vi "TAT_Com_PLC.vi"() -> ()   [LabVIEW 2017]
uses:
  Controls/PLC_Comm_State.ctl
  <vilib>/NI/Modbus Library/API/Master/Modbus Master.lvclass
  C:/Program Files (x86)/National Instruments/LabVIEW 2017/vi.lib/NI/Modbus Library/API/Modbus API.lvclass
  <vilib>/NI/Modbus Library/API/Wrapper/Create TCP Master.vi
  Global/PLC_to_Auto.vi
  <vilib>/NI/Modbus Library/API/Modbus API.lvclass
  <vilib>/NI/Modbus Library/API/Wrapper/API Main.lvlib
panel:
  out "register values":u16[](array[numeric])
  out "Array 2":u16[](array[numeric])
  out "PREVIOUS STATE":T1
  out "PLC IP Address":string
  out "error out 2":errorcluster
  out "error IO":errorcluster
  in  "stop 2":bool
  out "PLC STATUS station 2":bool
  out "LIVE":errorcluster
  out "Latch Error Case":errorcluster
  in  "error in":errorcluster
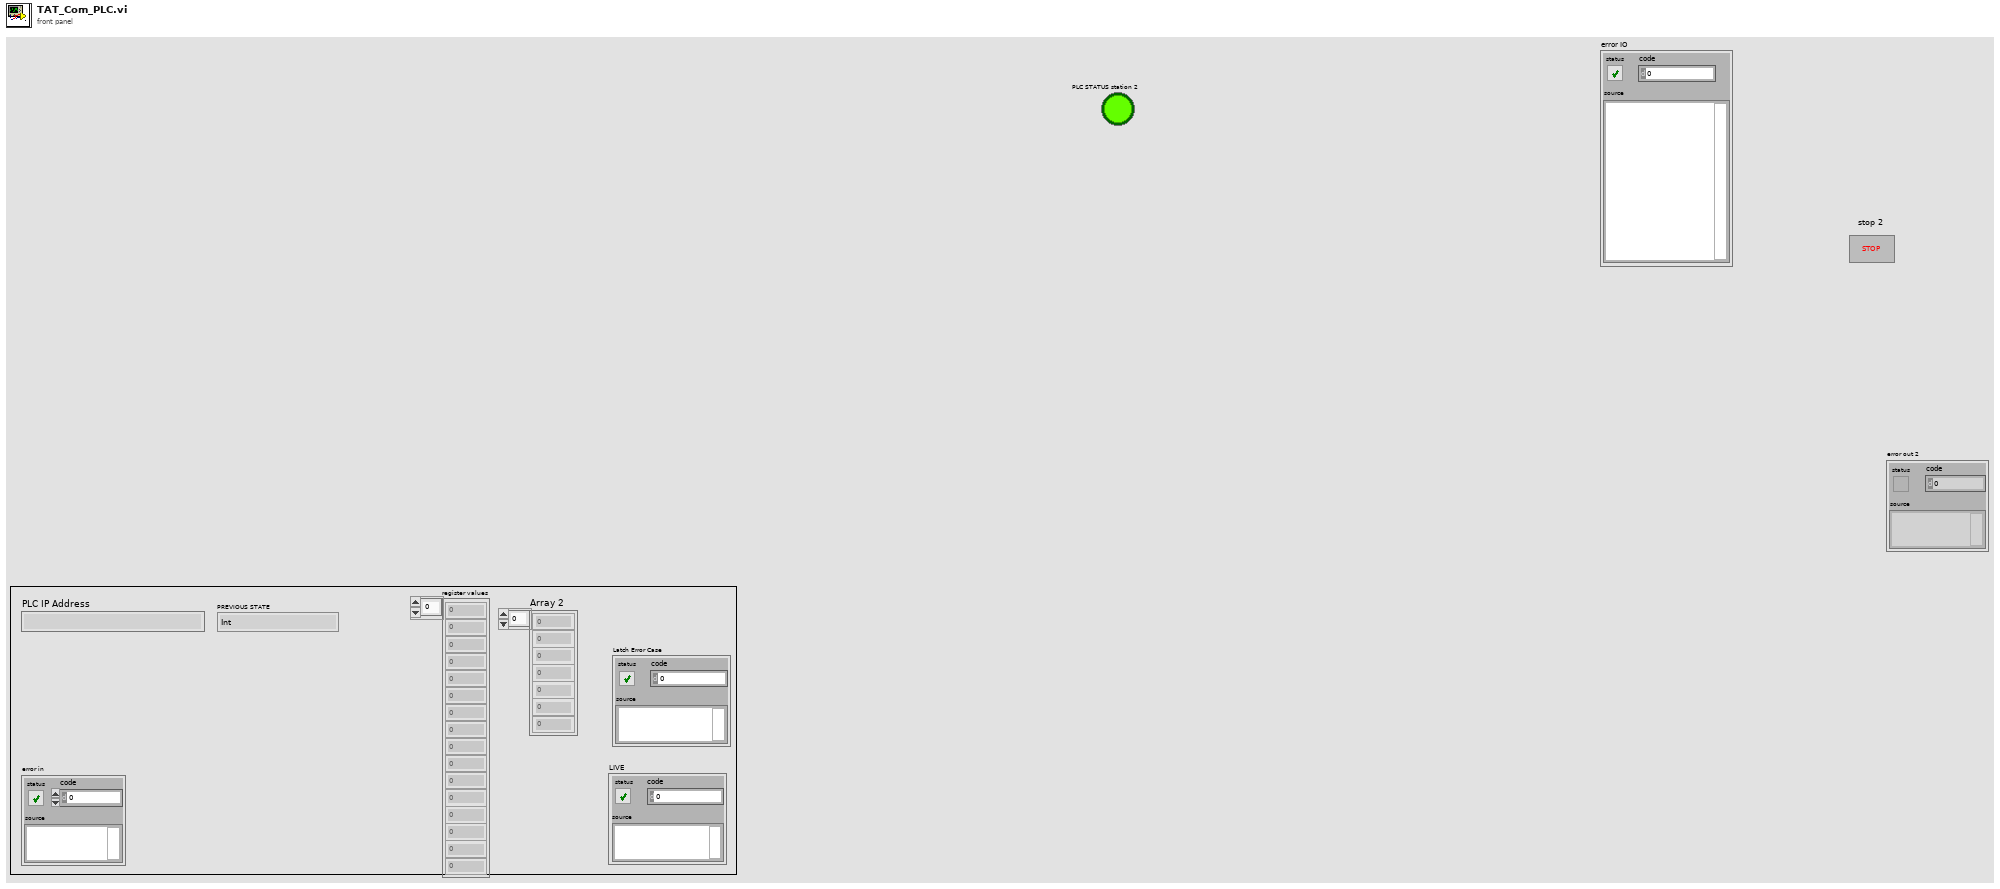
[diagram p1: front panel]
types:
  T1 = typedef "PLC_Comm_State.ctl" = enum16{"Int", "Connect", "Write", "Write2", "Write3", "Read", "Read2", "Read3", "Error", "Disconnect"}
  T2 = cluster{"PLC IP ADDRESS":string, "SCAN 1 COM":refnum<visa-resource-name>, "SCAN 2 COM":refnum<visa-resource-name>, "LOAD CELL COM":refnum<visa-resource-name>, "PRINTER IP ADDRESS":string}
  T3 = enum32{"invalid app kind", "Development System", "Run Time System", "Student Edition", "Embedded LabVIEW", "Evaluation", "Custom"}
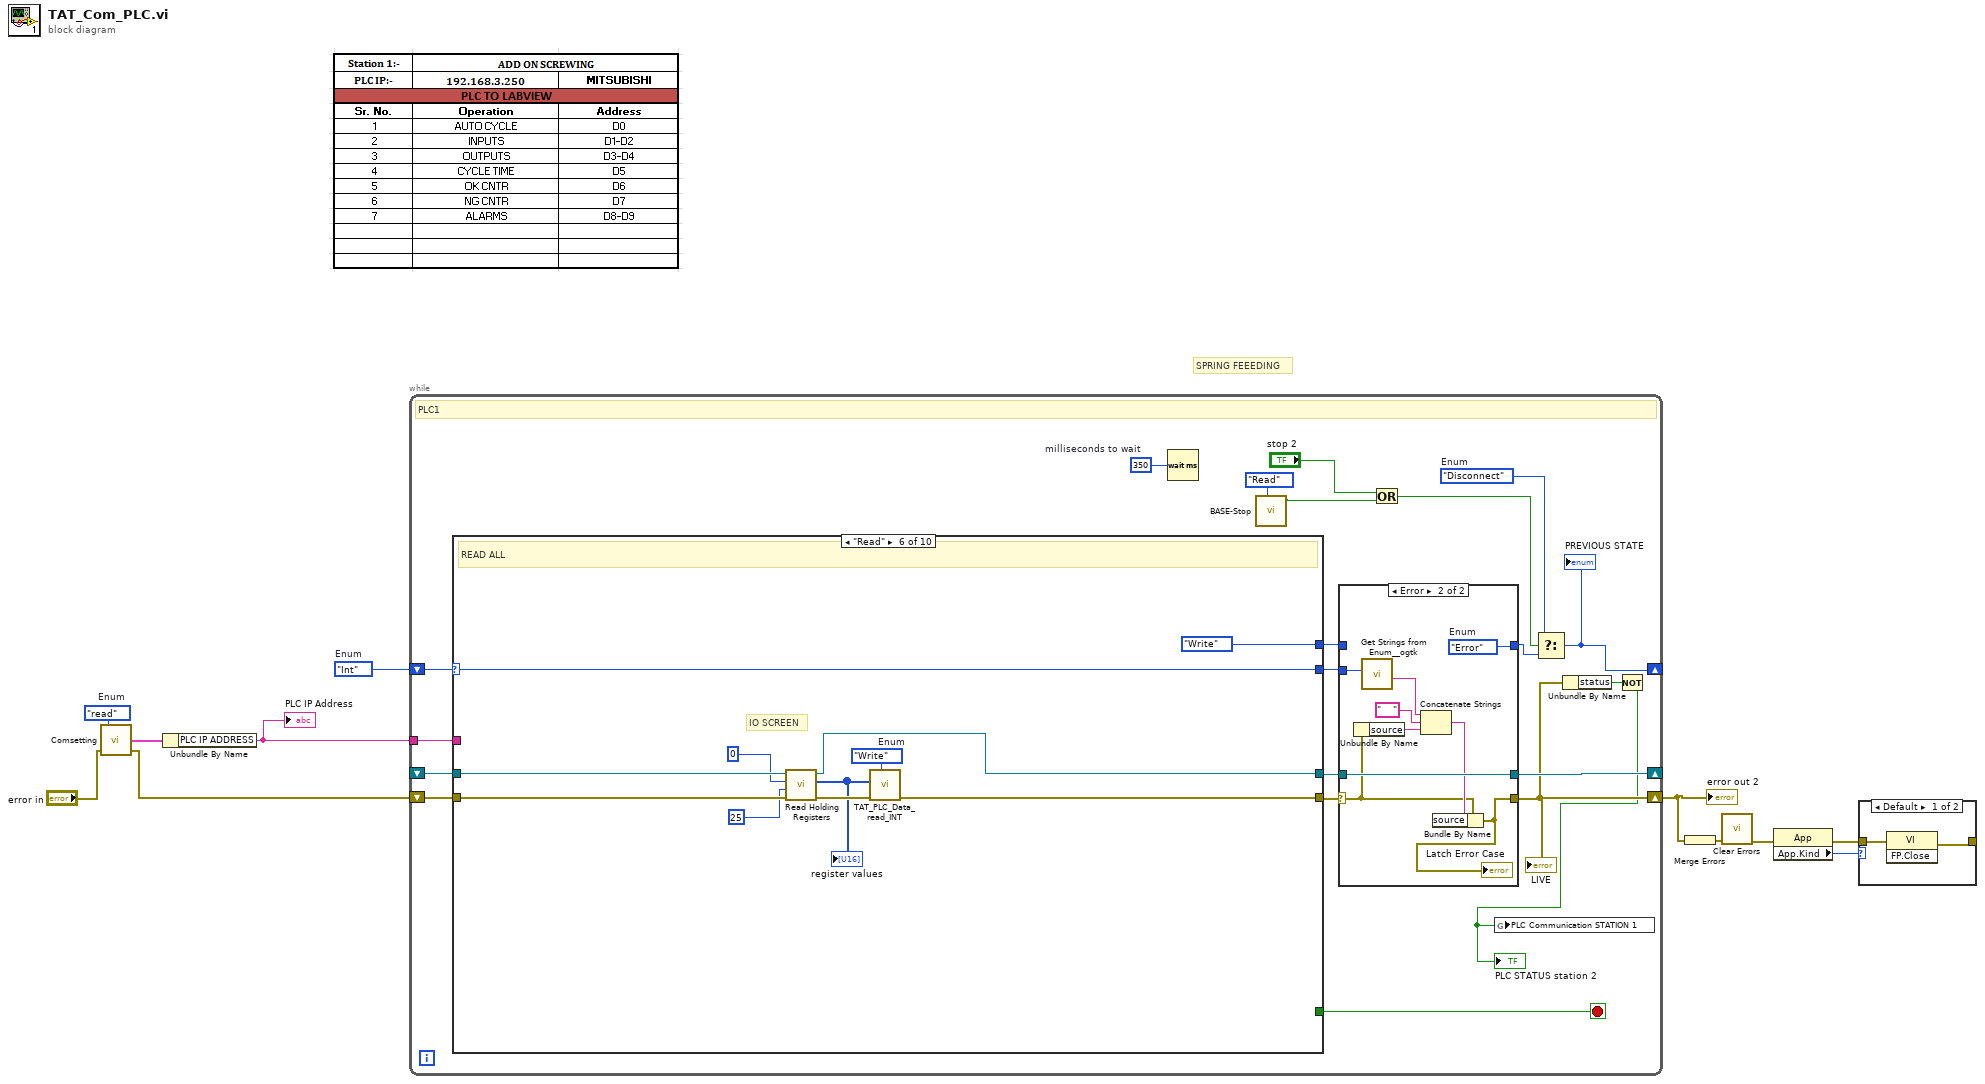
[diagram p0: block diagram]
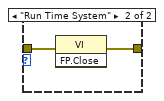
[diagram p2: hidden frame]
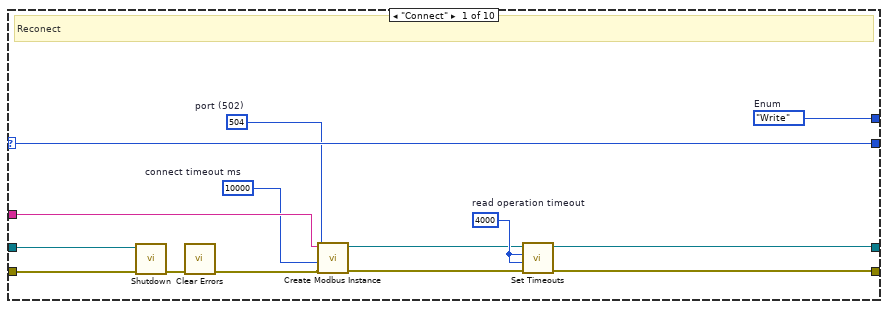
[diagram p4: hidden frame]
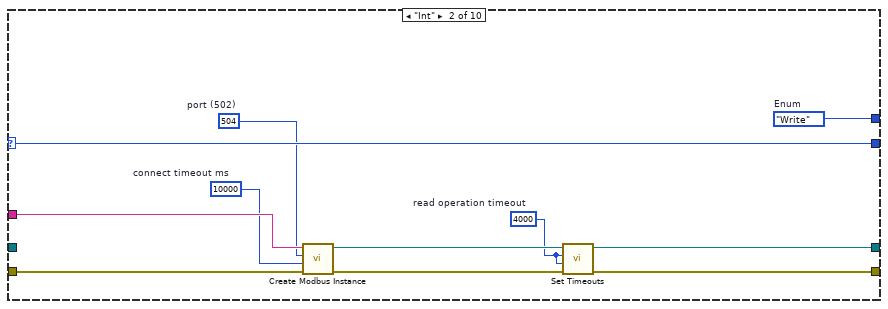
[diagram p5: hidden frame]
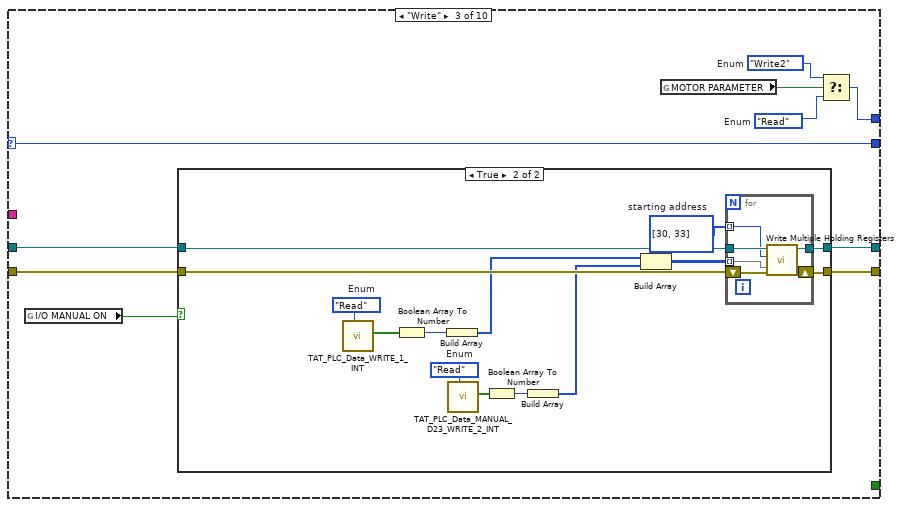
[diagram p6: hidden frame]
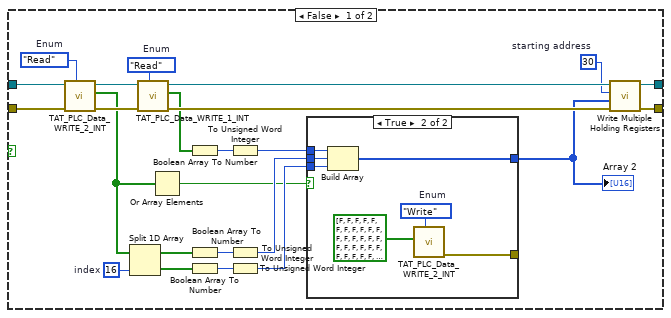
[diagram p7: hidden frame]
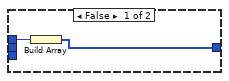
[diagram p8: hidden frame]
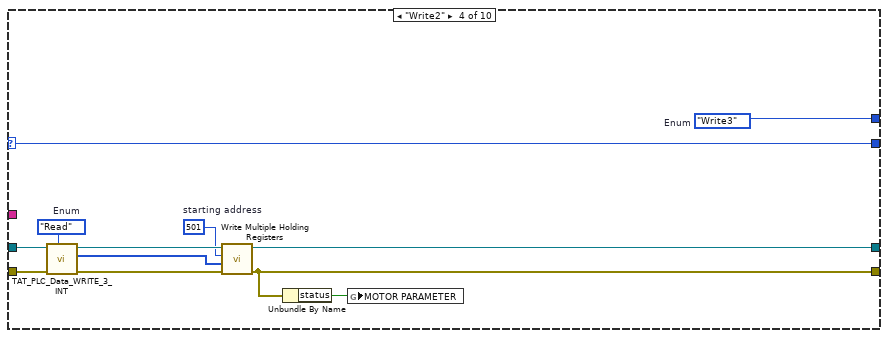
[diagram p9: hidden frame]
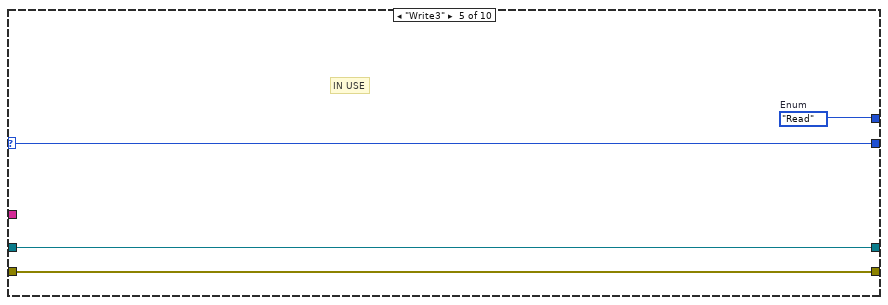
[diagram p10: hidden frame]
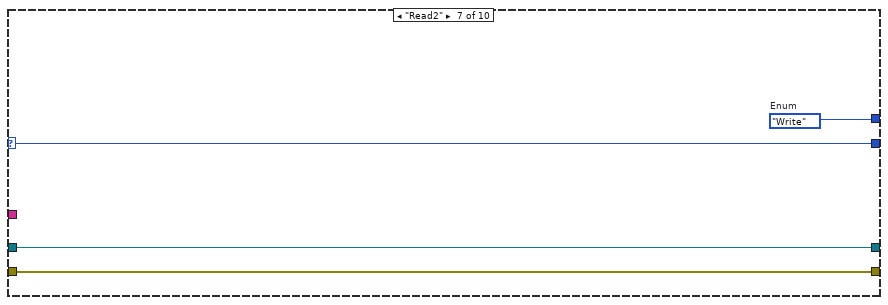
[diagram p11: hidden frame]
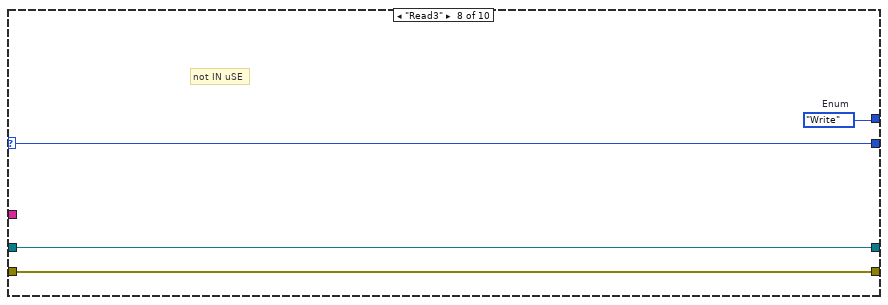
[diagram p12: hidden frame]
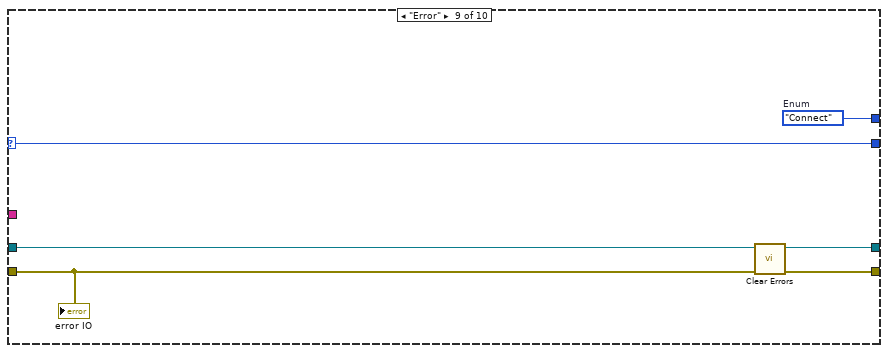
[diagram p13: hidden frame]
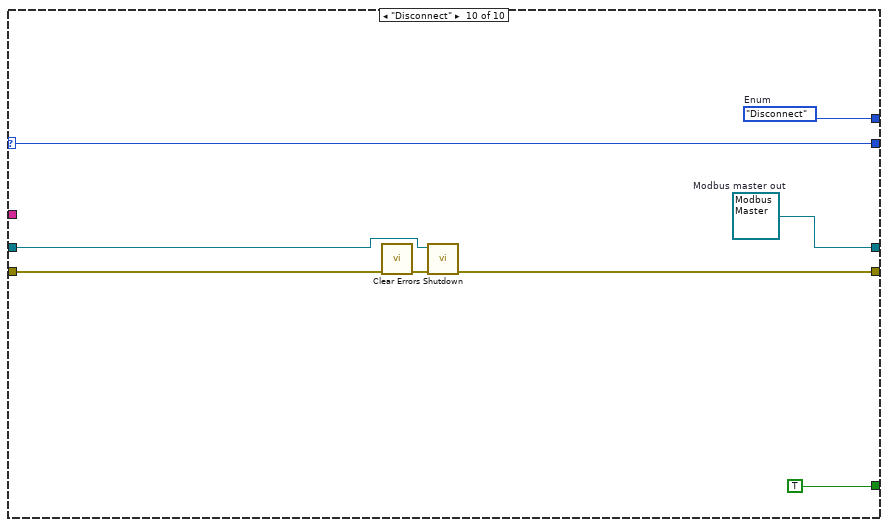
[diagram p14: hidden frame]
diagram:
  w4 = enum16{"read", "write"}."read"  # Enum
  w11 = PLC_Comm_State."Int"  # Enum
  # "SPRING FEEEDING"
  n1 = call "Comsetting.vi"("error in"="error in", "Enum"=w4) -> ("error our"=w1:errorcluster, "HardwareSetting"=w3:T2)  [unwired: 1 in, 1 out]
  n2 = Unbundle By Name(w3) -> ("PLC IP ADDRESS"=w5:string)
  "PLC IP Address" <- w5
  n3 = while {
    shift-right: [w23] -> _
    shift-left: w11 -> [w31]
    shift-right: [w18] -> w6
    shift-left: w1 -> [w30]
    shift-right: [w26] -> _
    shift-left: _ -> [w29]
    tunnel: w5 -> [w28]
    stop <- w24 stop-if-true
    w12 = u32 350  # milliseconds to wait
    w16 = PLC_Comm_State."Disconnect"  # Enum
    # "PLC1"
    n4 = case shown="\"Read\"" w31 {
      selector: w31 -> [w58 w68 w79 w141 w144 w156 w159 w161 w167 w175]
      tunnel: [w47 w60 w75 w132 w142 w153 w157 w164 w168 w172] -> w32
      tunnel: [w46 w62 w76 w135 w143 w152 w158 w163 w169 w170] -> w25
      tunnel: w30 -> [w54 w69 w78 w138 w142 w155 w157 w164 w165 w177]
      tunnel: w29 -> [w52 _ w77 w136 w143 w154 w158 w163 w169 w171]
      tunnel: w28 -> [w55 w66 _ _ _ _ _ _ _ _]
      tunnel: [w57 w67 w70 w140 w145 PLC_Comm_State."Write" ("Enum") w160 w162 w166 w174] -> w27
      tunnel: [_ _ _ _ _ _ _ _ _ TRUE] -> w24
      tunnel: [w58 w68 w79 w141 w144 w156 w159 w161 w167 w175] -> w21
      frame "Connect" {
        w49 = 4000  # read operation timeout
        w50 = u16 504  # port (502)
        w51 = 10000  # connect timeout ms
        w57 = PLC_Comm_State."Write"  # Enum
        # "Reconect"
        n5 = call-dynamic "Shutdown.vi"("error in"=w54, "Modbus instance in"=w52) -> ("error out"=w53:errorcluster)  [unwired: 9 in]
        n6 = call <vilib>:"Clear Errors.vi"("error in (no error)"=w53) -> ("error out"=w56:errorcluster)  [unwired: 5 in, 1 out]
        n7 = call-poly <vilib>:"Create Modbus Instance.vi"("error in"=w56, "connect timeout ms"=w51, "port (502)"=w50, "address"=w55) -> ("error out"=w48:errorcluster, "TCP master instance"=w45:refnum<class "Modbus Master.lvclass">)  [unwired: 6 in]
        n8 = call <vilib>:"Set Timeouts.vi"("error in"=w48, "write operation timeout"=w49, "read operation timeout"=w49, "Modbus master in"=w45) -> ("error out"=w47:errorcluster, "Modbus master out"=w46:refnum<class "Modbus Master.lvclass">)  [unwired: 6 in]
      }
      frame "Int" {
        w59 = 4000  # read operation timeout
        w64 = u16 504  # port (502)
        w65 = 10000  # connect timeout ms
        w67 = PLC_Comm_State."Write"  # Enum
        n9 = call-poly <vilib>:"Create Modbus Instance.vi"("error in"=w69, "connect timeout ms"=w65, "port (502)"=w64, "address"=w66) -> ("error out"=w61:errorcluster, "TCP master instance"=w63:refnum<class "Modbus Master.lvclass">)  [unwired: 6 in]
        n10 = call <vilib>:"Set Timeouts.vi"("error in"=w61, "write operation timeout"=w59, "read operation timeout"=w59, "Modbus master in"=w63) -> ("error out"=w60:errorcluster, "Modbus master out"=w62:refnum<class "Modbus Master.lvclass">)  [unwired: 6 in]
      }
      frame "Write" {
        w72 = PLC_Comm_State."Write2"  # Enum
        w71 = PLC_Comm_State."Read"  # Enum
        n11 = global read "PLC_to_Auto.vi" "I/O MANUAL ON"() -> (w74:bool)
        n12 = case shown="True" w74 {
          tunnel: w78 -> [w101 w121]
          tunnel: w77 -> [w100 w122]
          tunnel: [w99 w123] -> w76
          tunnel: [w82 w124] -> w75
          frame False {
            w89 = 16  # index
            w90 = enum16{"Read", "Write"}."Read"  # Enum
            w96 = u16 30  # starting address
            w97 = enum16{"Read", "Write"}."Read"  # Enum
            n13 = call "TAT_PLC_Data_WRITE_2_INT.vi"("Enum"=w90, "error in (no error)"=w101) -> ("error out"=w91:errorcluster, "Array 2"=w81:bool[])  [unwired: 8 in]
            n14 = Split 1D Array(array=w81, index=w89) -> (first subarray=w86:bool[], second subarray=w85:bool[])
            n15 = call "TAT_PLC_Data_WRITE_1_INT.vi"("Enum"=w97, "error in (no error)"=w91) -> ("error out"=w98:errorcluster, "Array 2"=w95:bool[])  [unwired: 8 in]
            n16 = Or Array Elements(Boolean array=w81) -> (logical OR=w80:bool)
            n17 = Boolean Array To Number(Boolean array=w95) -> (number=w94:u32)
            n18 = Boolean Array To Number(Boolean array=w86) -> (number=w88:u32)
            n19 = Boolean Array To Number(Boolean array=w85) -> (number=w87:u32)
            n20 = To Unsigned Word Integer(number=w94) -> (unsigned 16bit integer=w92:u16)
            n21 = To Unsigned Word Integer(number=w88) -> (unsigned 16bit integer=w84:u16)
            n22 = To Unsigned Word Integer(number=w87) -> (unsigned 16bit integer=w83:u16)
            n23 = case shown="True" w80 {
              tunnel: [w102 w105] -> w93
              tunnel: w92 -> [w103 w110]
              tunnel: w84 -> [_ w109]
              tunnel: w83 -> [_ w108]
              tunnel: [_ w104] -> _
              frame False {
                n24 = Build Array(w103) -> (w102:u16[])
              }
              frame True {
                w107 = enum16{"Read", "Write"}."Write"  # Enum
                n25 = Build Array(w110, w109, w108) -> (w105:u16[])
                n26 = call "TAT_PLC_Data_WRITE_2_INT.vi"("Enum"=w107, "Array"=bool[] [FALSE, FALSE, FALSE, FALSE, FALSE, FALSE, FALSE, FALSE, FALSE, FALSE, FALSE, FALSE, FALSE, FALSE, FALSE, FALSE, FALSE, FALSE, FALSE, FALSE, FALSE, FALSE, FALSE, FALSE, FALSE, FALSE, FALSE, FALSE, FALSE, FALSE, FALSE, FALSE]) -> ("error out"=w104:errorcluster)  [unwired: 8 in, 1 out]
              }
            }
            "Array 2" <- w93
            n27 = call-dynamic "Write Multiple Holding Registers.vi"("error in"=w98, "registers to write"=w93, "starting address"=w96, "Modbus instance in"=w100) -> ("error out"=w82:errorcluster, "Modbus instance out"=w99:refnum<class "Modbus API.lvclass">)  [unwired: 6 in]
          }
          frame True {
            w112 = enum16{"Read", "Write"}."Read"  # Enum
            w118 = enum16{"Read", "Write"}."Read"  # Enum
            w120 = u16[] [30, 33]  # starting address
            n28 = call "TAT_PLC_Data_WRITE_1_INT.vi"("Enum"=w112) -> ("Array 2"=w111:bool[])  [unwired: 9 in, 1 out]
            n29 = Boolean Array To Number(Boolean array=w111) -> (number=w119:u32)
            n30 = Build Array(w119) -> (w113:u32[])
            n31 = call "TAT_PLC_Data_MANUAL_D23_WRITE_2_INT.vi"("Enum"=w118) -> ("Array 2"=w117:bool[])  [unwired: 9 in, 1 out]
            n32 = Boolean Array To Number(Boolean array=w117) -> (number=w116:u32)
            n33 = Build Array(w116) -> (w114:u32[])
            n34 = Build Array(w113, w114) -> (w115:u32[][])
            n35 = for {
              tunnel: [w129] -> w123
              tunnel: w122 -> [w128]
              tunnel: w120 -> [w126] mode=indexing
              shift-right: [w130] -> w124
              shift-left: w121 -> [w127]
              tunnel: w115 -> [w125] mode=indexing
              n36 = call-dynamic "Write Multiple Holding Registers.vi"("error in"=w127, "registers to write"=w125, "starting address"=w126, "Modbus instance in"=w128) -> ("error out"=w130:errorcluster, "Modbus instance out"=w129:refnum<class "Modbus API.lvclass">)  [unwired: 6 in]
            }
          }
        }
        n37 = global read "PLC_to_Auto.vi" "MOTOR PARAMETER"() -> (w73:bool)
        n38 = Select(t=w72, s=w73, f=w71) -> (s? t:f=w70:T1)
      }
      frame "Write2" {
        w134 = u16 501  # starting address
        w139 = enum16{"Read", "Write"}."Read"  # Enum
        w140 = PLC_Comm_State."Write3"  # Enum
        n39 = call "TAT_PLC_Data_WRITE_3_INT.vi"("Enum"=w139, "error in (no error)"=w138) -> ("error out"=w137:errorcluster, "Array 2"=w133:u16[])  [unwired: 8 in]
        n40 = call-dynamic "Write Multiple Holding Registers.vi"("error in"=w137, "registers to write"=w133, "starting address"=w134, "Modbus instance in"=w136) -> ("error out"=w132:errorcluster, "Modbus instance out"=w135:refnum<class "Modbus API.lvclass">)  [unwired: 6 in]
        n41 = Unbundle By Name(w132) -> ("status"=w131:bool)
        n42 = global write "PLC_to_Auto.vi" "MOTOR PARAMETER"(w131) -> ()
      }
      frame "Write3" {
        w145 = PLC_Comm_State."Read"  # Enum
        # "IN USE"
      }
      frame "Read" {
        w150 = enum16{"Read", "Write"}."Write"  # Enum
        # "IO SCREEN"
        # "READ ALL"
        n43 = call-dynamic "Read Holding Registers.vi"("error in"=w155, "number of inputs"=u16 25 ("Numeric"), "starting address"=u16 0 ("Numeric"), "Modbus instance in"=w154) -> ("error out"=w149:errorcluster, "register values"=w148:u16[], "Modbus instance out"=w152:refnum<class "Modbus API.lvclass">)  [unwired: 5 in]
        "register values" <- w148
        n44 = call "TAT_PLC_Data_read_INT.vi"("Enum"=w150, "error in (no error)"=w149, "Array"=w148) -> ("error out"=w153:errorcluster)  [unwired: 7 in, 1 out]
      }
      frame "Read2" {
        w160 = PLC_Comm_State."Write"  # Enum
      }
      frame "Read3" {
        w162 = PLC_Comm_State."Write"  # Enum
        # "not IN uSE"
      }
      frame "Error" {
        w166 = PLC_Comm_State."Connect"  # Enum
        n45 = call <vilib>:"Clear Errors.vi"("error in (no error)"=w165) -> ("error out"=w168:errorcluster)  [unwired: 5 in, 1 out]
        "error IO" <- w165
      }
      frame "Disconnect" {
        w170 = refnum<class "Modbus Master.lvclass"> refnum  # Modbus master out
        w174 = PLC_Comm_State."Disconnect"  # Enum
        n46 = call <vilib>:"Clear Errors.vi"("error in (no error)"=w177) -> ("error out"=w173:errorcluster)  [unwired: 5 in, 1 out]
        n47 = call-dynamic "Shutdown.vi"("error in"=w173, "Modbus instance in"=w171) -> ("error out"=w172:errorcluster)  [unwired: 9 in]
      }
    }
    n48 = Wait (ms)(milliseconds to wait=w12) -> ()  [unwired: 1 out]
    n49 = call "BASE-Stop.vi"("Enum"=enum16{"Read", "Write"}."Read") -> ("Stop"=w14:bool)  [unwired: 10 in]
    n50 = case shown="Error" w32 {
      selector: w32 -> [w35 w38]
      tunnel: [w35 w36] -> w18
      tunnel: [w34 w37] -> w22
      tunnel: w27 -> [w34 _]
      tunnel: [w33 w44] -> w26
      tunnel: w25 -> [w33 w44]
      tunnel: w21 -> [_ w42]
      frame No Error {
      }
      frame Error {
        w37 = PLC_Comm_State."Error"  # Enum
        n51 = Unbundle By Name(w38) -> ("source"=w43:string)
        n52 = call <userlib>:"Get Strings from Enum__ogtk.vi"("Enum"=w42) -> ("String Value"=w41:string)  [unwired: 7 in, 3 out]
        n53 = Concatenate Strings(w41, "    " ("string"), w43) -> (w39:string)
        n54 = Bundle By Name(cluster=w38, "source"=w39) -> (w36:errorcluster)
        "Latch Error Case" <- w36
      }
    }
    "LIVE" <- w18
    n55 = Or(x="stop 2", y=w14) -> (x .or. y?=w20:bool)
    n56 = Select(t=w16, s=w20, f=w22) -> (s? t:f=w23:T1)
    "PREVIOUS STATE" <- w23
    n57 = Unbundle By Name(w18) -> ("status"=w19:bool)
    n58 = Not(x=w19) -> (.not. x?=w13:bool)
    "PLC STATUS station 2" <- w13
    n59 = global write "PLC_to_Auto.vi" "PLC Communication STATION 1"(w13) -> ()
  }
  "error out 2" <- w6
  n60 = Merge Errors(w6) -> (w10:errorcluster)
  n61 = call <vilib>:"Clear Errors.vi"("error in (no error)"=w10) -> ("error out"=w9:errorcluster)  [unwired: 5 in, 1 out]
  n62 = property class="App"(error in=w9) -> (error out=w8:errorcluster, "App.Kind"=w7:T3)  [unwired: 1 in, 1 out]
  n63 = case shown="Default" w7 {
    tunnel: w8 -> [w179 w181]
    tunnel: [w178 w180] -> _
    frame Default {
      n64 = invoke class="VI" method="FP.Close"(error in=w179) -> (error out=w178:errorcluster)  [unwired: 2 in, 2 out]
    }
    frame "Run Time System" {
      n65 = invoke class="VI" method="FP.Close"(error in=w181) -> (error out=w180:errorcluster)  [unwired: 2 in, 2 out]
    }
  }
